vi "Read Default Value.vi"(8 "error in (no error)":errorcluster, 11 "Numeric Data Type in":refnum<class "Numeric Data Type.lvclass">) -> (0 "error out":errorcluster, 2 "Default Value":string, 3 "Numeric Data Type out":refnum<class "Numeric Data Type.lvclass">)   [LabVIEW 2018, in "Numeric Data Type.lvclass"]
uses:
  Numeric Data Type.lvclass
  Numeric Data Type.lvclass/Numeric Data Type.ctl
  Complex Number to String (CXT).vi
  Complex Number to String (CDB).vi
  Complex Number to String (CSG).vi
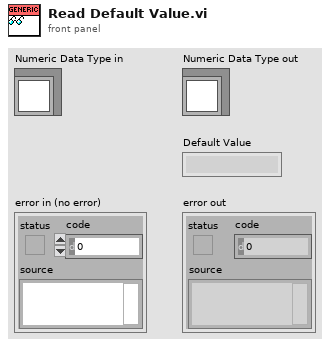
[diagram p1: front panel]
types:
  T1 = typedef "Numeric Data Type.lvclass/Representation Enum.ctl" = enum16{"Extended (EXT)", "Double (DBL)", "Single (SGL)", "Fixed-Point (FXP)", "Quad Integer (I64)", "Long Integer (I32)", "Word Integer (I16)", "Byte Integer (I8)", "Unsigned Quad (U64)", "Unsigned Long (U32)", "Unsigned Word (U16)", "Unsigned Byte (U8)", "Complex Extended (CXT)", "Complex Double (CDB)", "Complex Single (CSG)"}
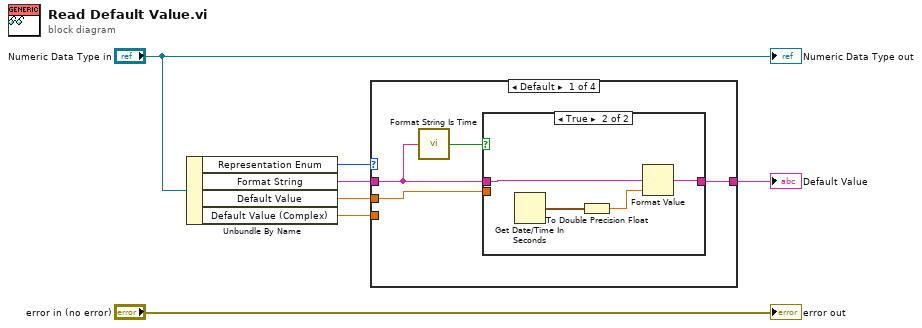
[diagram p0: block diagram]
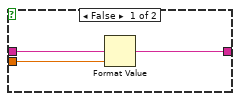
[diagram p2: hidden frame]
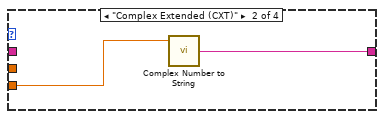
[diagram p3: hidden frame]
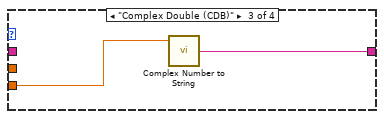
[diagram p4: hidden frame]
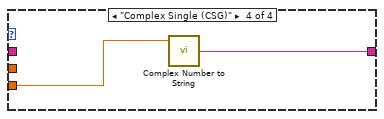
[diagram p5: hidden frame]
diagram:
  n1 = Unbundle By Name("Numeric Data Type in") -> ("Representation Enum"=w4:T1, "Format String"=w3:string, "Default Value"=w5:dbl, "Default Value (Complex)"=w1:cdb)
  n2 = case shown="Default" w4 {
    tunnel: w5 -> [w11 _ _ _]
    tunnel: w3 -> [w9 _ _ _]
    tunnel: [w10 w20 w22 w24] -> w2
    tunnel: w1 -> [_ w19 w21 w23]
    frame Default {
      n3 = call "Format String Is Time.vi"("Format String"=w9) -> ("Time?"=w8:bool)
      n4 = case shown="True" w8 {
        tunnel: w11 -> [w14 _]
        tunnel: [w13 w16] -> w10
        tunnel: w9 -> [w12 w18]
        frame False {
          n5 = Format Value(format string=w12, value (0)=w14) -> (output string=w13:string)  [unwired: 1 in]
        }
        frame True {
          n6 = Get Date/Time In Seconds() -> (seconds since 1Jan1904=w17:timestamp)
          n7 = To Double Precision Float(number=w17) -> (double precision float=w15:dbl)
          n8 = Format Value(format string=w18, value (0)=w15) -> (output string=w16:string)  [unwired: 1 in]
        }
      }
    }
    frame "Complex Extended (CXT)" {
      n9 = call-poly "Complex Number to String.vi"("number"=w19) -> ("Complex-format string"=w20:string)  [unwired: 3 in]
    }
    frame "Complex Double (CDB)" {
      n10 = call-poly "Complex Number to String.vi"("number"=w21) -> ("Complex-format string"=w22:string)  [unwired: 3 in]
    }
    frame "Complex Single (CSG)" {
      n11 = call-poly "Complex Number to String.vi"("number"=w23) -> ("Complex-format string"=w24:string)  [unwired: 3 in]
    }
  }
  "Default Value" <- w2
  "error out" <- "error in (no error)"
  "Numeric Data Type out" <- "Numeric Data Type in"
